vi "PCO_SetCmosLineExposureDelay.vi"(8 "error in (no error)":errorcluster {"code" format="%x"}, 9 "dwDelayLines":u32, 10 "dwExposureLines":u32, 11 "ph":u64) -> (0 "error out":errorcluster {"code" format="%x"}, 2 "ErrorMessage":i32 format="%x", 3 "ph out":u64)   [LabVIEW 2019, in "SDK.lvlib" / "SpecialCommandsEdge.lvlib"]
doc: "<b>Description:</b>\nThis function sets the exposure and delay line settings for the Lightsheet scanning mode. It is only available when Lightsheet scanning mode has been successfully enabled by PCO_SetCmosLineTiming.\n\n<b>Supported camera type:</b>\npco.edge with Camera Link interface\n\n<b>Descriptor dependency:</b>\nNone"
uses:
  SpecialCommandsEdge.lvlib
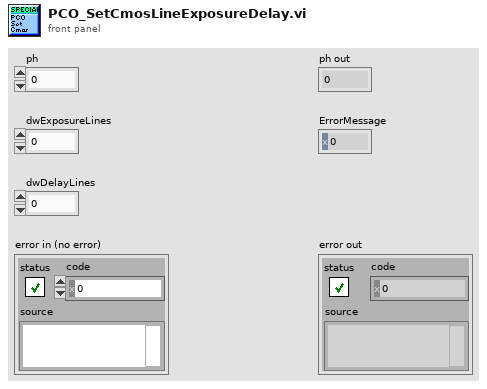
[diagram p1: front panel]
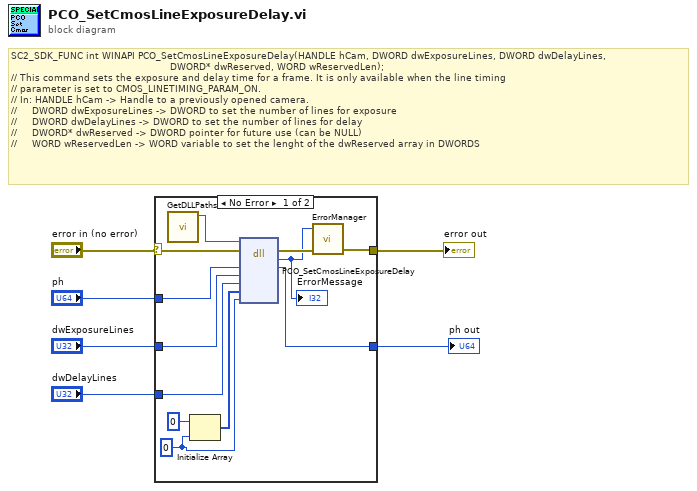
[diagram p0: block diagram]
diagram:
  # "SC2_SDK_FUNC int WINAPI PCO_SetCmosLineExposureDelay(HANDLE hCam, DWORD dwExposureLines, DWORD dwDelayLines,\n                                                     DWORD* dwReserved, WORD wReservedLen);\n// This command sets the exposure and delay time for a frame. It is only available when the line timing \n// parameter is set to CMOS_LINETIMING_PARAM_ON.\n// In: HANDLE hCam -> Handle to a previously opened camera.\n//     DWORD dwExposureLines -> DWORD to set the number of lines for exposure\n//     DWORD dwDelayLines -> DWORD to set the number of lines for delay\n//     DWORD* dwReserved -> DWORD pointer for future use (can be NULL)\n//     WORD wReservedLen -> WORD variable to set the lenght of the dwReserved array in DWORDS"
  n1 = case shown="No Error" "error in (no error)" {
    selector: "error in (no error)" -> [w11 w20]
    tunnel: "ph" -> [w18 w19]
    tunnel: [w17 w19] -> w5
    tunnel: "dwExposureLines" -> [w16 _]
    tunnel: "dwDelayLines" -> [w15 _]
    tunnel: [w9 w20] -> w2
    frame No Error {
      w12 = u16 0 ("dimension size")
      n2 = call "GetDLLPaths.vi"() -> ("SC2_Cam_Path"=w7:path)  [unwired: 9 in, 2 out]
      n3 = Initialize Array(u32 0, w12) -> (w13:u32[])
      n4 = dll-call lib="?" fn="PCO_SetCmosLineExposureDelay"(path in=w7, error in=w11, "ph"=w18, "dwExposureLines"=w16, "dwDelayLines"=w15, "dwReserved"=w13, "wReservedLen"=w12) -> (error out=w10:errorcluster, "return type"=w8:i32, "ph"=w17:u64)  [unwired: 5 in, 1 out]
      "ErrorMessage" <- w8
      n5 = call "ErrorManager.vi"("error in (no error)"=w10, "error code"=w8) -> ("error out"=w9:errorcluster)  [unwired: 3 in]
    }
    frame Error {
    }
  }
  "ph out" <- w5
  "error out" <- w2
